vi "Write Addr.vi"(8 "error in (no error)":errorcluster, 10 "Addr":refnum<visa-resource-name>, 11 "Lakeshore 331 in":refnum<class "Lakeshore 331.lvclass">) -> (0 "error out":errorcluster, 3 "Lakeshore 331 out":refnum<class "Lakeshore 331.lvclass">)   [LabVIEW 2022 SP3, in "Lakeshore 331.lvclass"]
uses:
  Lakeshore 331.lvclass
  Lakeshore 331.lvclass/Lakeshore 331.ctl
  Temp Control.lvclass
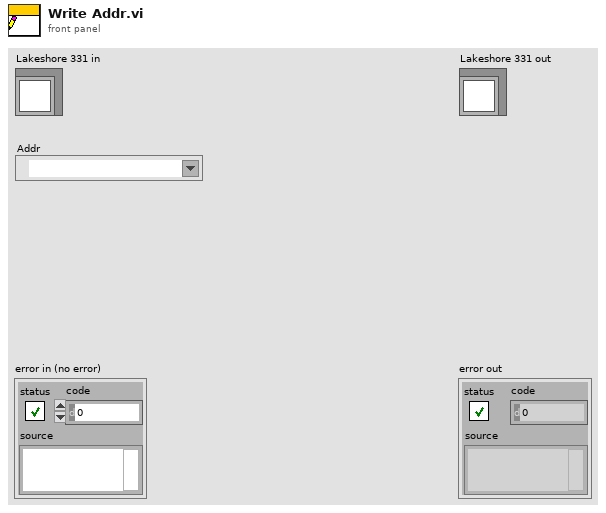
[diagram p1: front panel]
types:
  T1 = typedef "Lakeshore 331.lvclass/Lakeshore 331 Settings.ctl" = cluster{"Addr":refnum<visa-resource-name>, "Ch Prefix":string, "Ch Select":i32[]}
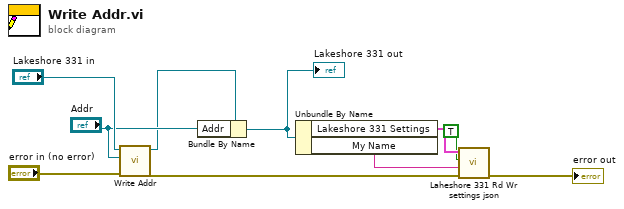
[diagram p0: block diagram]
diagram:
  n1 = call-parent "Write Addr.vi"("error in (no error)"="error in (no error)", "Addr"="Addr", "Temp Control in"="Lakeshore 331 in") -> ("error out"=w4:errorcluster, "Temp Control out"=w7:refnum<class "Lakeshore 331.lvclass">)  [unwired: 7 in]
  n2 = Bundle By Name(cluster=w7, "Addr"="Addr") -> (w6:refnum<class "Lakeshore 331.lvclass">)
  "Lakeshore 331 out" <- w6
  n3 = Unbundle By Name(w6) -> ("Lakeshore 331 Settings"=w5:T1, "My Name"=w1:string)
  n4 = call "Laheshore 331 Rd Wr settings json.vi"("error in (no error)"=w4, "section"=w1, "Write? (F:Read)"=TRUE, "Lakeshore 331 Settings"=w5) -> ("error out"=→"error out":errorcluster)  [unwired: 6 in, 1 out]
